vi "FER(9600).vi"(7 "Поток с  декодера\nВитерби":bool[](array[boolean])) -> (8 "Нет синхр!":bool)   [LabVIEW 2017]
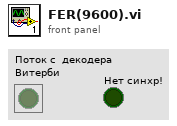
[diagram p1: front panel]
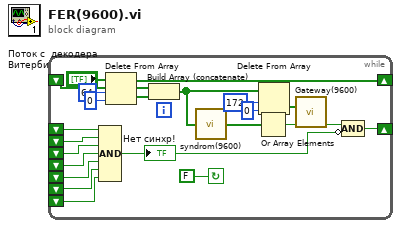
[diagram p0: block diagram]
diagram:
  n1 = while {
    shift-right: [w14] -> _
    shift-left: _ -> [w13]
    shift-right: [w7] -> _
    shift-left: _ -> [w12]
    shift-left: _ -> [w11]
    shift-left: _ -> [w10]
    shift-left: _ -> [w9]
    shift-left: _ -> [w8]
    shift-left: _ -> [w5]
    shift-left: _ -> [w4]
    stop <- FALSE continue-if-true
    n2 = Compound Arithmetic op=AND(w12, w11, w10, w9, w8, w5, w4) -> (w6:bool)
    "Нет синхр!" <- w6
    n3 = Delete From Array(array="Поток с  декодера\nВитерби", length=64, index=0) -> (deleted portion=w15:bool[], array with subset deleted=w14:bool[])
    n4 = Build Array (concatenate)(w13, w15) -> (w3:bool[])
    n5 = call "syndrom(9600).vi"("Кадр для  вычисления \nсиндрома"=w3) -> ("Синдром"=w19:bool[])  [unwired: 14 in]
    n6 = Or Array Elements(Boolean array=w19) -> (logical OR=w2:bool)
    n7 = Delete From Array(array=w3, length=172, index=0) -> (deleted portion=w1:bool[])  [unwired: 1 out]
    n8 = call "Gateway(9600).vi"("Принятый кадр"=w1, "Ошибка"=w2) -> ()  [unwired: 14 in]
    n9 = Compound Arithmetic op=AND(w2, invert w6) -> (w7:bool)
  }
